vi "Mac.vi"(8 "error in (no error)":errorcluster, 10 "Font in":string, 11 "Font":refnum<vi>) -> (0 "error out":errorcluster, 2 "Font out":string)   [LabVIEW 2021]
uses:
  <vilib>/LabVIEW Icon API/lv_icon/lv_icon.lvlib
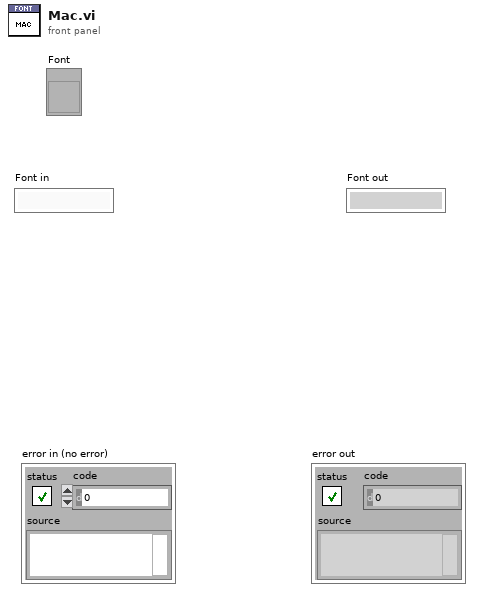
[diagram p1: front panel]
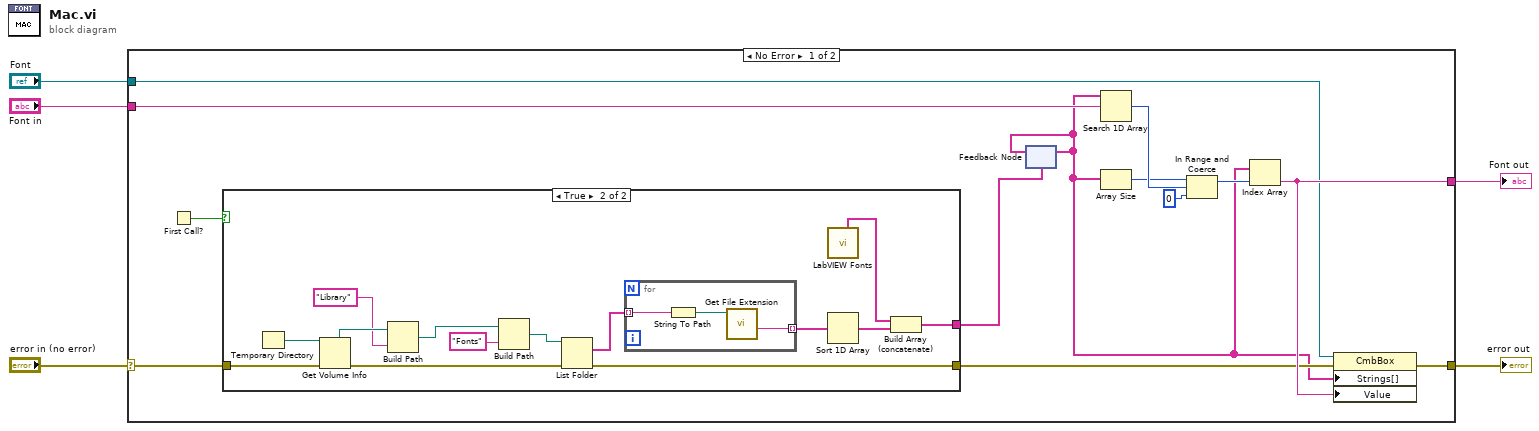
[diagram p0: block diagram]
diagram:
  n1 = case shown="No Error" "error in (no error)" {
    selector: "error in (no error)" -> [w18 w38]
    tunnel: [w17 w38] -> w4
    tunnel: "Font in" -> [w12 w37]
    tunnel: [w11 w37] -> w2
    tunnel: "Font" -> [w10 _]
    frame No Error {
      n2 = First Call?() -> (First Call?: T/F=w8:bool)
      n3 = case shown="True" w8 {
        tunnel: w18 -> [w19 w28]
        tunnel: [_ w22] -> w7
        tunnel: [w19 w20] -> w9
        frame False {
        }
        frame True {
          n4 = Temporary Directory() -> (w33:path)
          n5 = Get Volume Info(8:w28, 11:w33) -> (0:w26:errorcluster, 5:w32:path)  [unwired: 4 out]
          n6 = Build Path(base path=w32, name or relative path="Library") -> (appended path=w29:path)
          n7 = Build Path(base path=w29, name or relative path="Fonts") -> (appended path=w27:path)
          n8 = List Folder(path=w27, error in=w26) -> (filenames=w25:string[], error out=w20:errorcluster)  [unwired: 4 out]
          n9 = for {
            tunnel: w25 -> [w36] mode=indexing
            tunnel: [w34] -> w24 mode=indexing
            n10 = String To Path(string=w36) -> (path=w35:path)
            n11 = call <vilib>:"Get File Extension.vi"("file"=w35) -> ("filename without extension"=w34:string)  [unwired: 1 in, 9 out]
          }
          n12 = call <vilib>:"LabVIEW Fonts.vi"() -> ("Additional Fonts"=w21:string[])  [unwired: 1 in, 10 out]
          n13 = Sort 1D Array(array=w24) -> (sorted array=w23:string[])
          n14 = Build Array (concatenate)(w21, w23) -> (w22:string[])
        }
      }
      n15 = feedback #1(w7) -> (w6:string[])
      n16 = feedback-in #1(w6) -> ()
      n17 = Search 1D Array(1D array=w6, element=w12) -> (index of element=w16:i32)  [unwired: 1 out]
      n18 = Array Size(array=w6) -> (size(s)=w13:i32)
      n19 = In Range and Coerce(upper limit=w13, x=w16, lower limit=0 ("x")) -> (coerced(x)=w14:i32)  [unwired: 1 out]
      n20 = Index Array(array=w6, index=w14) -> (element=w11:string)
      n21 = property class="CmbBox"(reference=w10, error in=w9, "Strings[]"=w6, "Value"=w11) -> (error out=w17:errorcluster)  [unwired: 1 out]
    }
    frame Error {
    }
  }
  "error out" <- w4
  "Font out" <- w2
